vi "Init DaqEngine local DI SM.vi"(7 "DI TaskName":string, 8 "error in (no error)":errorcluster, 11 "DAQ Process AppData":T1) -> (0 "error out":errorcluster, 1 "local LoopCmdQ":refnum<queue>, 3 "DAQProcess DI AppData+":T10)   [LabVIEW 2017, in "DAQ.lvclass"]
doc: "Developed by Kevin Thompson\nkevin@thompsonengineering.net\n\nCopyright 2018-2020\nThompson Engineering, LLC"
uses:
  DAQ.lvclass
  Process_DAQ SM AppData--cluster.ctl
  DataTypes/TD DAQ Settings--cluster.ctl
  DataTypes/TD DI Instrument Settings--cluster.ctl
  DataTypes/TD AI Instrument Settings--cluster.ctl
  DataTypes/TD AI InstSettings--cluster.ctl
  TD SimAI Ranges--cluster.ctl
  <vilib>/TELLC/Dynamic CVT API/TD Dynamic CVT DVR--ref.ctl
  DataTypes/TD DI local thread params--clustser.ctl
  TD local raw DI Data--cluster.ctl
  DataTypes/TD DI TaskIO.ctl
  DAQ.lvclass/DAQ.ctl
  Accessors/Get DAQNodes Dict.vi
  Accessors/Get DAQ Settings.vi
  Get DI DAQ SMQ - single.vi
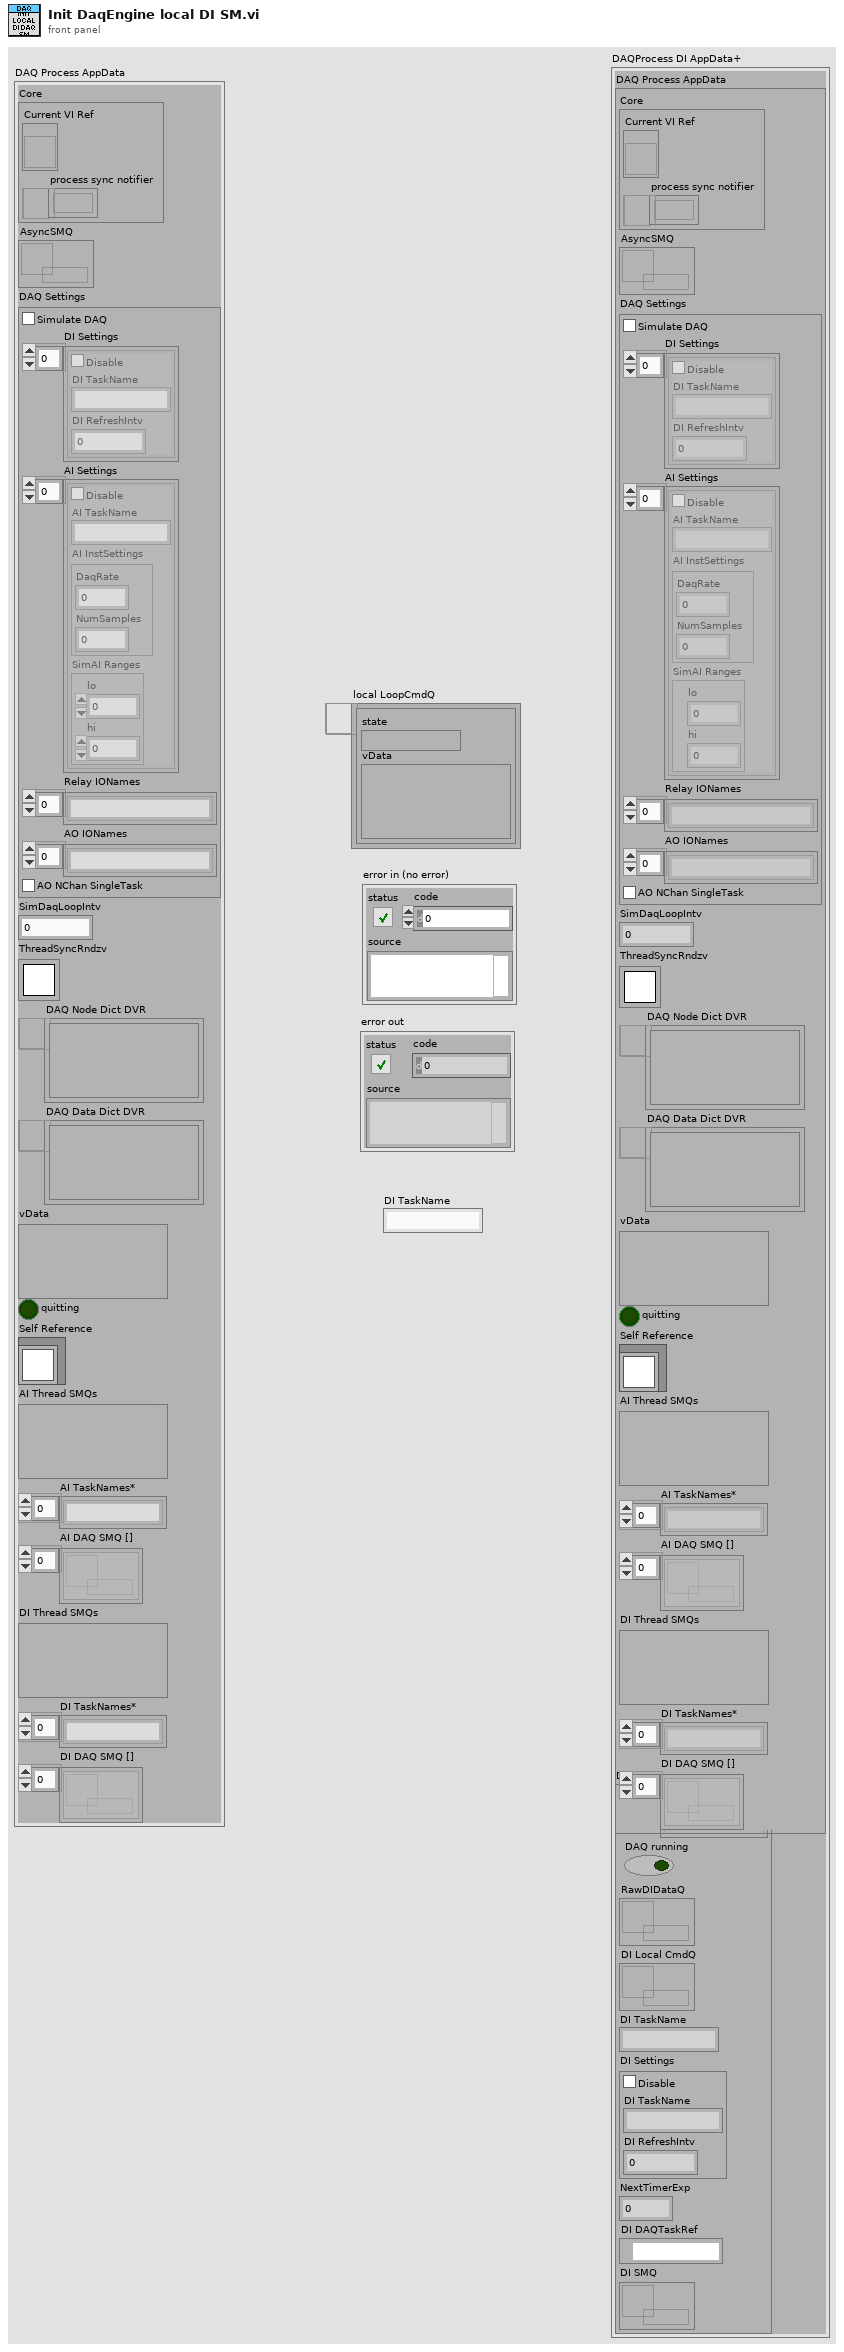
[diagram p1: front panel]
types:
  T1 = typedef "DAQ.lvclass/Process_DAQ SM AppData--cluster.ctl" = cluster{"Core":cluster{"Current VI Ref":refnum<vi>, "process sync notifier":refnum<notifier>}, "AsyncSMQ":refnum<queue>, "DAQ Settings":T2, "SimDaqLoopIntv":i32, "ThreadSyncRndzv":T7, "DAQ Node Dict DVR":T8, "DAQ Data Dict DVR":T8, "vData":variant, "quitting":bool, "Self Reference":refnum<class "DAQ.lvclass">, "AI Thread SMQs":variant, "AI TaskNames*":string[], "AI DAQ SMQ []":refnum<queue>[], "DI Thread SMQs":variant, "DI TaskNames*":string[], "DI DAQ SMQ []":refnum<queue>[]}
  T2 = typedef "DAQ.lvclass/TD DAQ Settings--cluster.ctl" = cluster{"Simulate DAQ":bool, "DI Settings":T3[], "AI Settings":T4[], "Relay IONames":string[], "AO IONames":string[], "AO NChan SingleTask":bool}
  T3 = typedef "DAQ.lvclass/TD DI Instrument Settings--cluster.ctl" = cluster{"Disable":bool, "DI TaskName":string, "DI RefreshIntv":i32}
  T4 = typedef "DAQ.lvclass/TD AI Instrument Settings--cluster.ctl" = cluster{"Disable":bool, "AI TaskName":string, "AI InstSettings":T5, "SimAI Ranges":T6}
  T5 = typedef "DAQ.lvclass/TD AI InstSettings--cluster.ctl" = cluster{"DaqRate":dbl, "NumSamples":i32}
  T6 = typedef "DAQ.lvclass/TD SimAI Ranges--cluster.ctl" = cluster{"lo":dbl, "hi":dbl}
  T7 = typedef "Rendezvous RefNum" = refnum<k1>
  T8 = typedef "TD Dynamic CVT DVR--ref.ctl" = refnum<data-value>
  T9 = typedef "DAQ.lvclass/TD DI local thread params--clustser.ctl" = cluster{"DI IONames":string[], "DAQ running":bool, "RawDIDataQ":refnum<queue>, "DI Local CmdQ":refnum<queue>, "DI TaskName":string, "DI Settings":T3, "NextTimerExp":dbl, "DI DAQTaskRef":refnum<k21>, "DI SMQ":refnum<queue>}
  T10 = cluster{"DAQ Process AppData":T1, "DI thread params":T9}
  T11 = typedef "DAQ.lvclass/TD DI TaskIO.ctl" = cluster{"DI TaskName":string, "IONames":string[], "DAQmxDI TaskRef":refnum<k21>}
  T12 = typedef "DAQ.lvclass/TD local raw DI Data--cluster.ctl" = cluster{dbl, "data":bool[]}
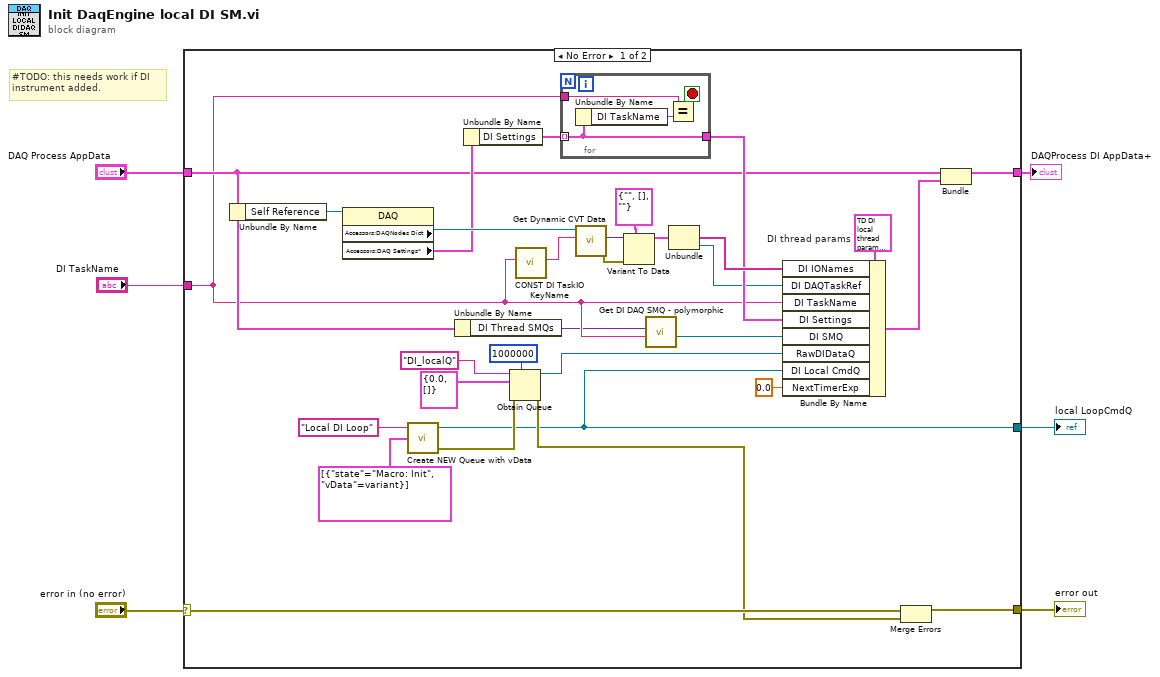
[diagram p0: block diagram]
diagram:
  # "#TODO: this needs work if DI\ninstrument added."
  n1 = case shown="No Error" "error in (no error)" {
    selector: "error in (no error)" -> [w35 w42]
    tunnel: "DAQ Process AppData" -> [w9 _]
    tunnel: [w30 _] -> w5
    tunnel: [w31 _] -> w2
    tunnel: [w36 w42] -> w4
    tunnel: "DI TaskName" -> [w8 _]
    frame No Error {
      w28 = T9 {"DI IONames"=[], "DAQ running"=FALSE, "RawDIDataQ"=refnum, "DI Local CmdQ"=refnum, "DI TaskName"="", "DI Settings"={"Disable"=FALSE, "DI TaskName"="", "DI RefreshIntv"=0}, "NextTimerExp"=0.0, "DI DAQTaskRef"="", "DI SMQ"=refnum}  # DI thread params
      n2 = Unbundle By Name(w9) -> ("Self Reference"=w24:refnum<class "DAQ.lvclass">)
      n3 = property class="DAQ"(reference=w24) -> ("Accessors:DAQNodes Dict"=w20:T8, "Accessors:DAQ Settings*"=w15:T2)  [unwired: 1 in, 2 out]
      n4 = call <vilib>:"Create NEW Queue with vData.vi"("Initial States"=cluster{"state":string, "vData":variant}[] [{"state"="Macro: Init", "vData"=variant}], "Name (SMQ)"="Local DI Loop") -> ("error out"=w34:errorcluster, "queue out"=w30:refnum<queue>)  [unwired: 2 in]
      n5 = Unbundle By Name(w9) -> ("DI Thread SMQs"=w7:variant)
      n6 = Unbundle By Name(w15) -> ("DI Settings"=w16:T3[])
      n7 = Obtain Queue(max queue size (-1, unlimited)=1000000, name (unnamed)="DI_localQ" ("format string"), element data type=T12 {0.0, "data"=[]} ("Raw DI Data"), error in (no error)=w34) -> (queue out=w26:refnum<queue>, error out=w33:errorcluster)  [unwired: 1 in, 1 out]
      n8 = call "CONST DI TaskIO KeyName.vi"("DI TaskName"=w8) -> ("DI TaskIO (KeyName)"=w19:string)  [unwired: 10 in]
      n9 = for {
        tunnel: w16 -> [w40] mode=indexing
        tunnel: w8 -> [w39]
        tunnel: [w40] -> w14
        stop <- w38 stop-if-true
        n10 = Unbundle By Name(w40) -> ("DI TaskName"=w41:string)
        n11 = Equal?(x=w39, y=w41) -> (x = y?=w38:bool)
      }
      n12 = call <vilib>:"Get Dynamic CVT Data.vi"("DataName"=w19, "dCVT DVR"=w20) -> ("error out"=w22:errorcluster, "value"=w21:variant)  [unwired: 6 in, 2 out]
      n13 = Variant To Data(error in=w22, type=T11 {"DI TaskName"="", "IONames"=[], "DAQmxDI TaskRef"=""} ("DI TaskIO"), Variant=w21) -> (data=w23:T11)  [unwired: 1 out]
      n14 = call-poly "Get DI DAQ SMQ - polymorphic.vi"("AI TaskName"=w8, "AI Thread SMQs"=w7) -> ("AI DAQ SMQ"=w10:refnum<queue>)  [unwired: 7 in, 2 out]
      n15 = Unbundle(w23) -> ("IONames"=w17:string[], "DAQmxDI TaskRef"=w11:refnum<k21>)  [unwired: 1 out]
      n16 = Bundle By Name(cluster=w28, "DI IONames"=w17, "DI DAQTaskRef"=w11, "DI TaskName"=w8, "DI Settings"=w14, "DI SMQ"=w10, "RawDIDataQ"=w26, "DI Local CmdQ"=w30, "NextTimerExp"=0.0) -> (w29:T9)
      n17 = Merge Errors(w35, w33) -> (w36:errorcluster)
      n18 = Bundle("DAQ Process AppData"=w9, "DI thread params"=w29) -> (w31:T10)  [unwired: 1 in]
    }
    frame Error {
    }
  }
  "error out" <- w4
  "local LoopCmdQ" <- w5
  "DAQProcess DI AppData+" <- w2
